vi "220428_snipper_v15.vi"(0 "Input picture 3":picture caption="Input", 1 "hh:mm:ss":T2={"left"=50, "top"=439, "right"=600, "bottom"=479} caption="input hh:mm:ss") -> (2 "4-bit pixmap":u8[][][](array[numeric]), 3 "sniped pic.":picture[](array[picture]), 4 "String N":i32, 5 "elapsed time(s)":dbl[][](array[numeric]) format="%#_3g")   [LabVIEW 2016]
panel:
  in  "Read data":bool
  out "Sumtime(s)":dbl
  out "From_TapN":dbl
  out "moveLog(Row, Col.) 2":i32[][](array[numeric])
  out "from TotalP 2":i32
  out "Out signal 2":bool
  out "From_TapN 2":dbl
  in  "N1 test(Col.)":i32
  in  "タブ制御器":T1(tab)
  out "Input picture":picture caption="Input"
  out "Void potition":cluster{"Y":dbl[], "Y":dbl[]}[](graph)
  out "Graph data":i32[][](array[numeric])
  out "Rawdata pixmap":u8[][](array[numeric]) caption="4ビットピックスマップ"
  in  "path to PNG file":path=path "G:/マイドライブ/STEPN/STEPN_walking/PNG/220510-220515/IMG_6679.PNG" caption="PNGファイルパス"
  out "Debug test pic. 4":picture caption="12 delete pic."
  out "Expand test pic. 5":picture caption="12 delete Expand pic."
  out "string(start,end) 2":i32[][](array[numeric])
  out "Debug test pic. 2":picture caption="7x pic."
  out "7x move(min, max)":i32[][](array[numeric])
  out "searchCol.by7x":i32[](array[numeric])
  out "ΔmoveLog(Row, Col.)":i32[][][](array[numeric])
  out "Debug test pic. 3":picture caption="Δ  pic."
  out "deruta bitmap":i32[][](array[numeric])
  out "OK/NG":string[][](array[string])
  out "Δ N":i32
  out "7xMove Log":i32[][][](array[numeric])
  out "NG_moveLog(Row, Col.)出力":i32[][][](array[numeric])
  out "OutPut_moveLog_all 2":i32[][][](array[numeric])
  out "2forward moveLog 2":i32[][][](array[numeric])
  out "7x Expand pic.":picture
  out "Δ Expand pic.":picture
  out "2F Expand pic.":picture
  out "pixmap size(T×Y)":i32[](array[numeric])
  out "Debug test pic.":picture caption="Debug naname pic."
  out "4-bit pixmap 3":u8[][](array[numeric])
  out "string 2":string[](array[string])
  out "To:finish Col. 2":i32
  out "to Total point 2":i32
  out "Left_TotalP 2":i32
  out "R_endCol. 2":i32
  out "L_endCol. 2":i32
  out "Debug test pic. 8":picture caption="Debug test pic."
  out "2forwardN 2":i32
  out "Right(1) or Left(2) 2":enum16{"1>2", "1=2", "1<2"}(ring)
  out "To(1) or From(2) 2":enum16{"1>2", "1=2", "1<2"}(ring)
  out "2forward totalP 2":i32[](array[numeric])
  out "Goal 2":i32
  out "from\\to 2":string
  out "Right_TotalP 2":i32
  out "Expand test pic. 2":picture caption="Debug naname pic."
  out "naname":bool
  out "Pixture size (Y, X)":i32[](array[numeric])
  out "naname_TotalP":i32
  out "TapN":dbl
  in  "naname hide":bool=TRUE
  out "4 detected":bool
  out "2F Expand pic. 2":picture caption="2F Expand pic."
  out "Δ Expand pic. 2":picture caption="Δ Expand Pic."
  out "2F Expand pic. 3":picture caption="2F Expand pic."
  out "R_TapN 2":dbl
  out "L_TapN 2":dbl
  out "Debug test pic. 6":picture caption="Debug test pic."
  out "Debug test pic. 7":picture caption="Debug test pic."
  out "Debug test pic. 5":picture caption="Debug test pic."
  in  "N1_test":bool
  # "v12 : 35/5(文字1のy/x) で切り取り\nv13 : 2段階①35/5で切り取り /一旦一区切り\n　　　　　　　　  ②2forward search(4を踏んだ時点で中断)"
  # "sec"
  # "%"
  # "0"
  # "1"
  # "2"
  # "3"
  # "4"
  # "5"
  # "6"
  # "7"
  # "Picture"
  # "File"
  # "OFF"
  # "ON"
  # "2forward : Yellow\nΔ　：Green"
  # "Left : blue\nTo : red"
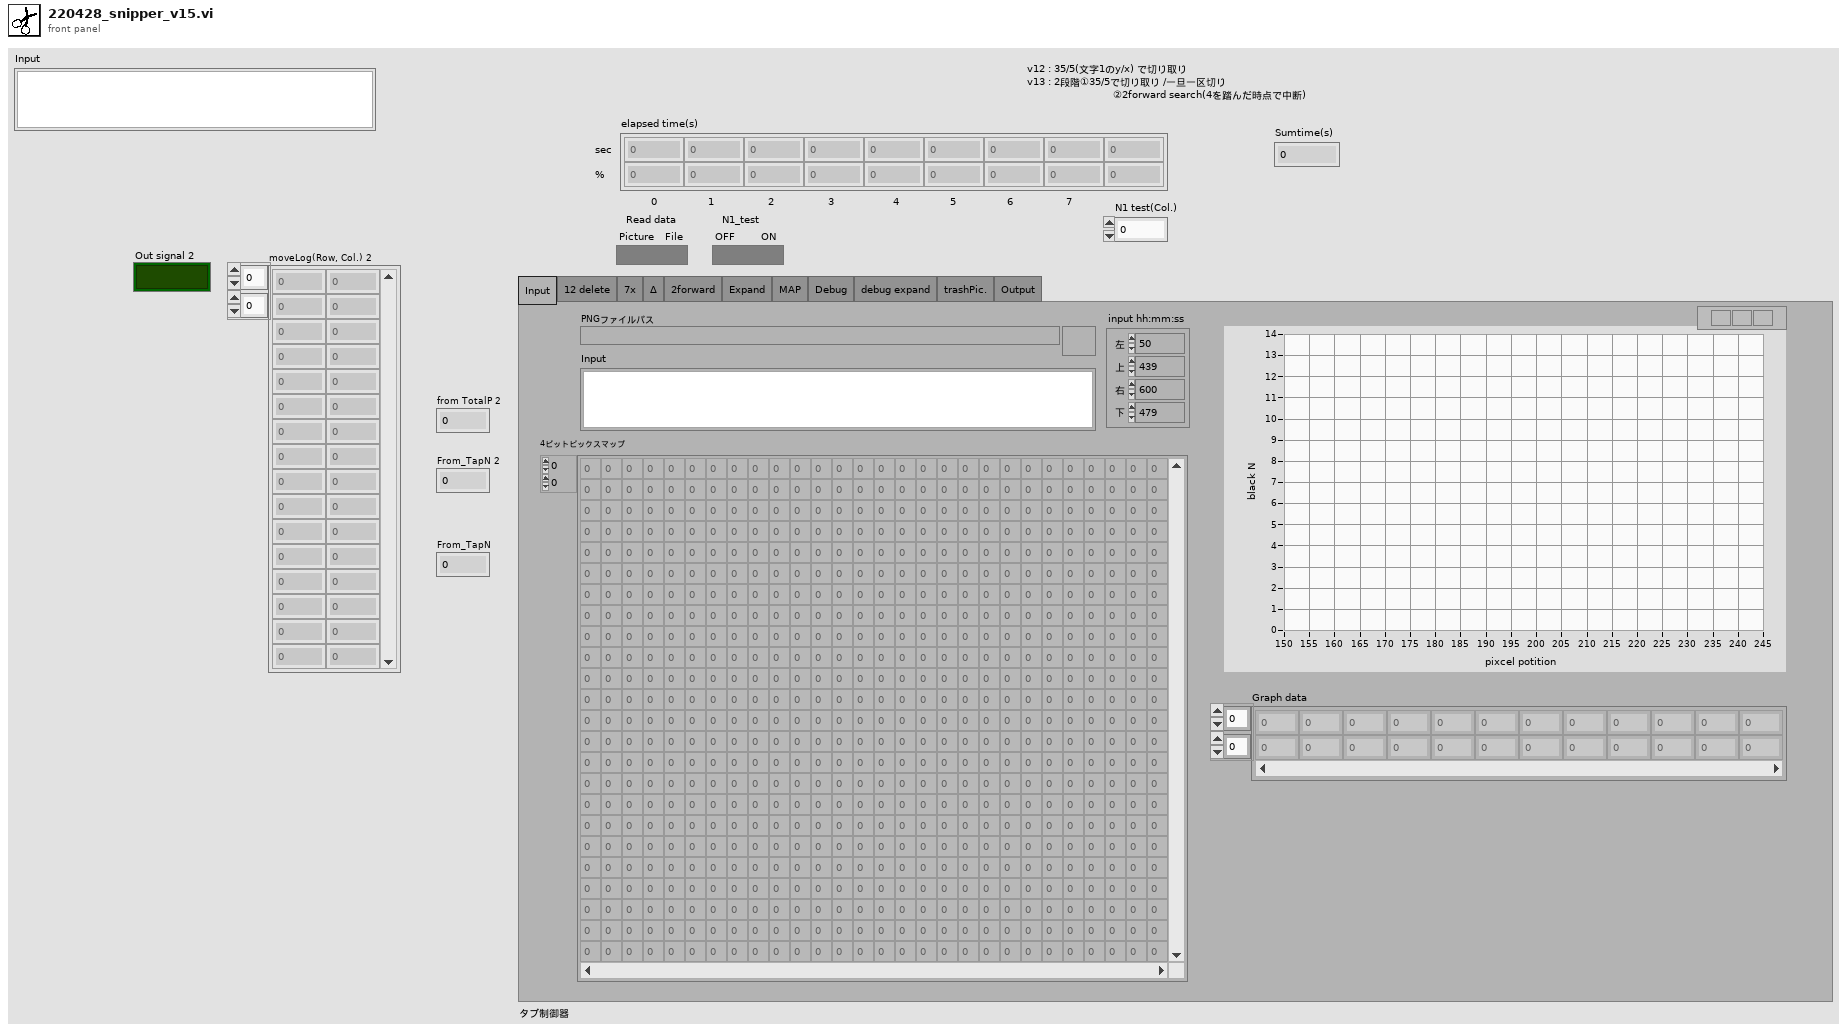
[diagram p1: front panel]
types:
  T1 = enum32{"Input", "12 delete", "7x", "Δ", "2forward", "Expand", "MAP", "Debug", "debug expand", "trashPic.", "Output"}
  T2 = cluster{"left":i16, "top":i16, "right":i16, "bottom":i16}
  T3 = typedef "imagedata.ctl" = cluster{"image type":i32, "image depth":i32, "image":u8[], "mask":u8[], "colors":u32[], "Rectangle":cluster{"left":i16, "top":i16, "right":i16, "bottom":i16}}
  T4 = typedef "LVBoundsTypeDef.ctl" = cluster{"Width":u32, "Height":u32}
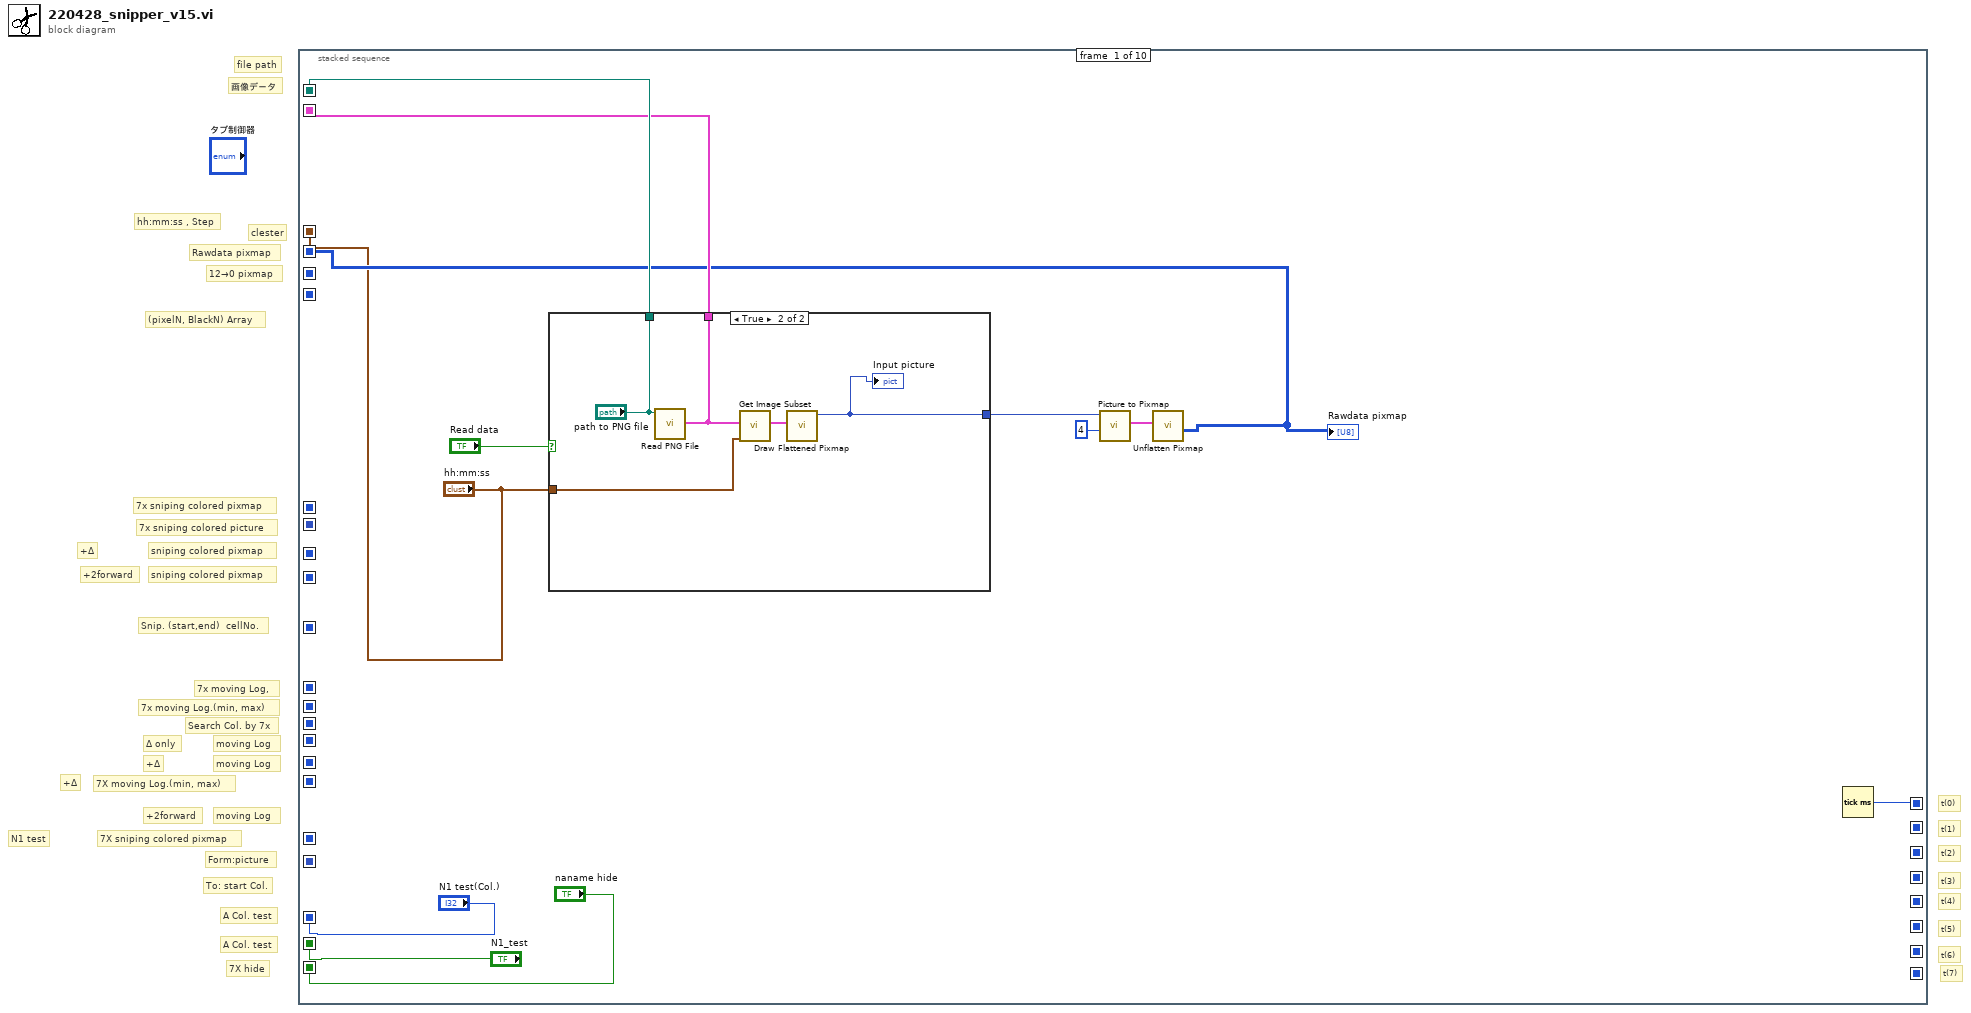
[diagram p0: block diagram]
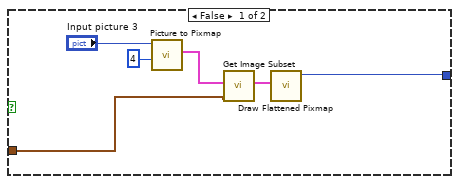
[diagram p2: hidden frame]
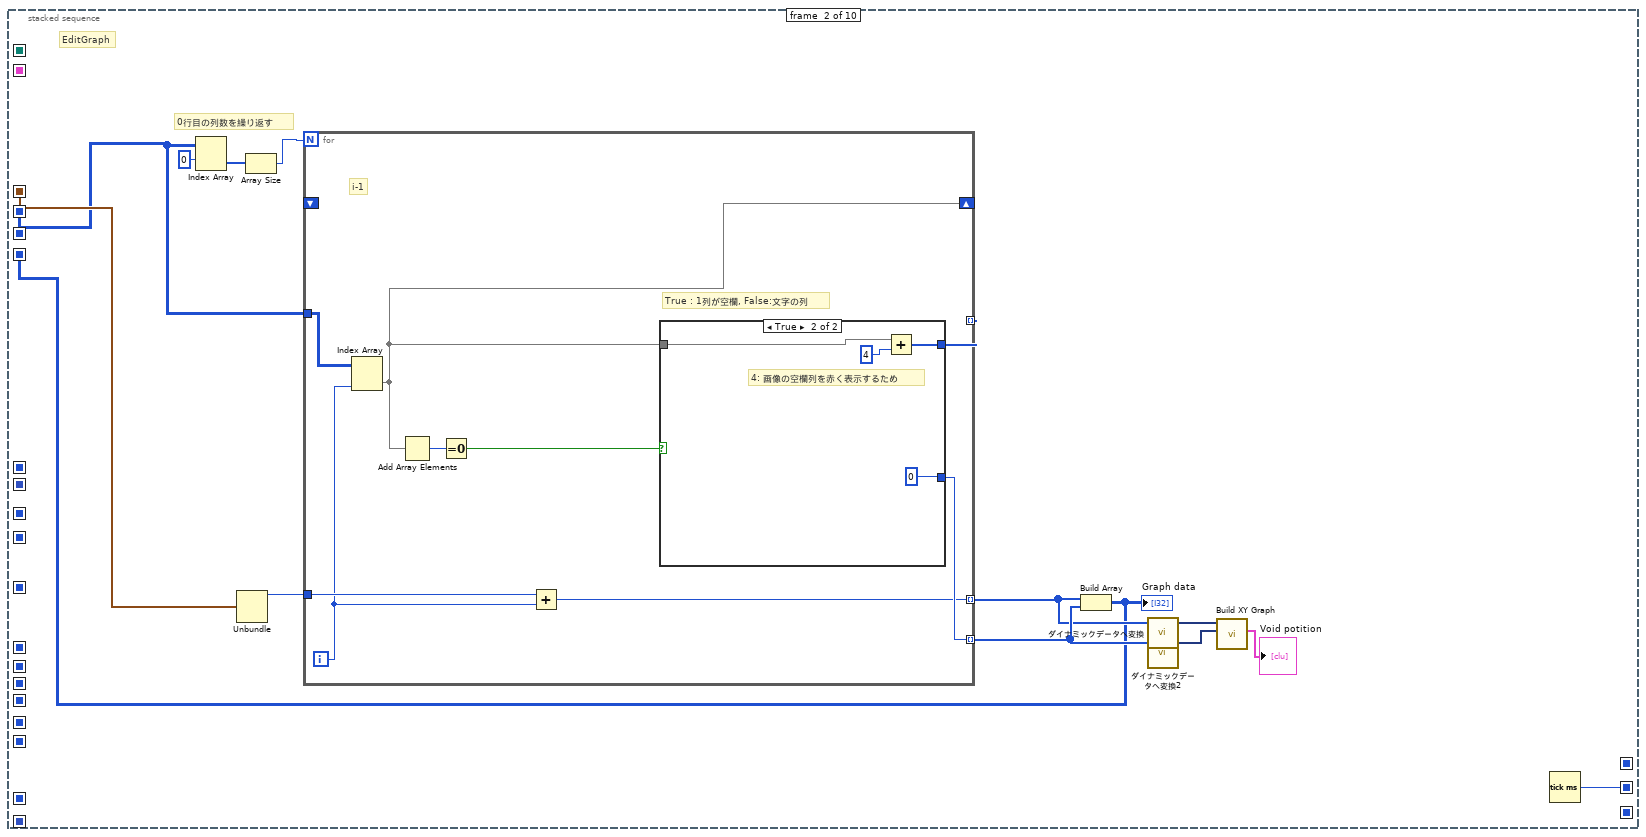
[diagram p3: hidden frame]
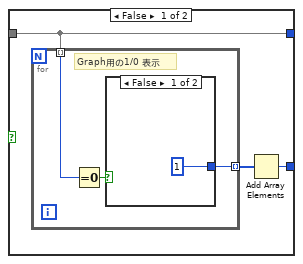
[diagram p4: hidden frame]
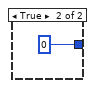
[diagram p5: hidden frame]
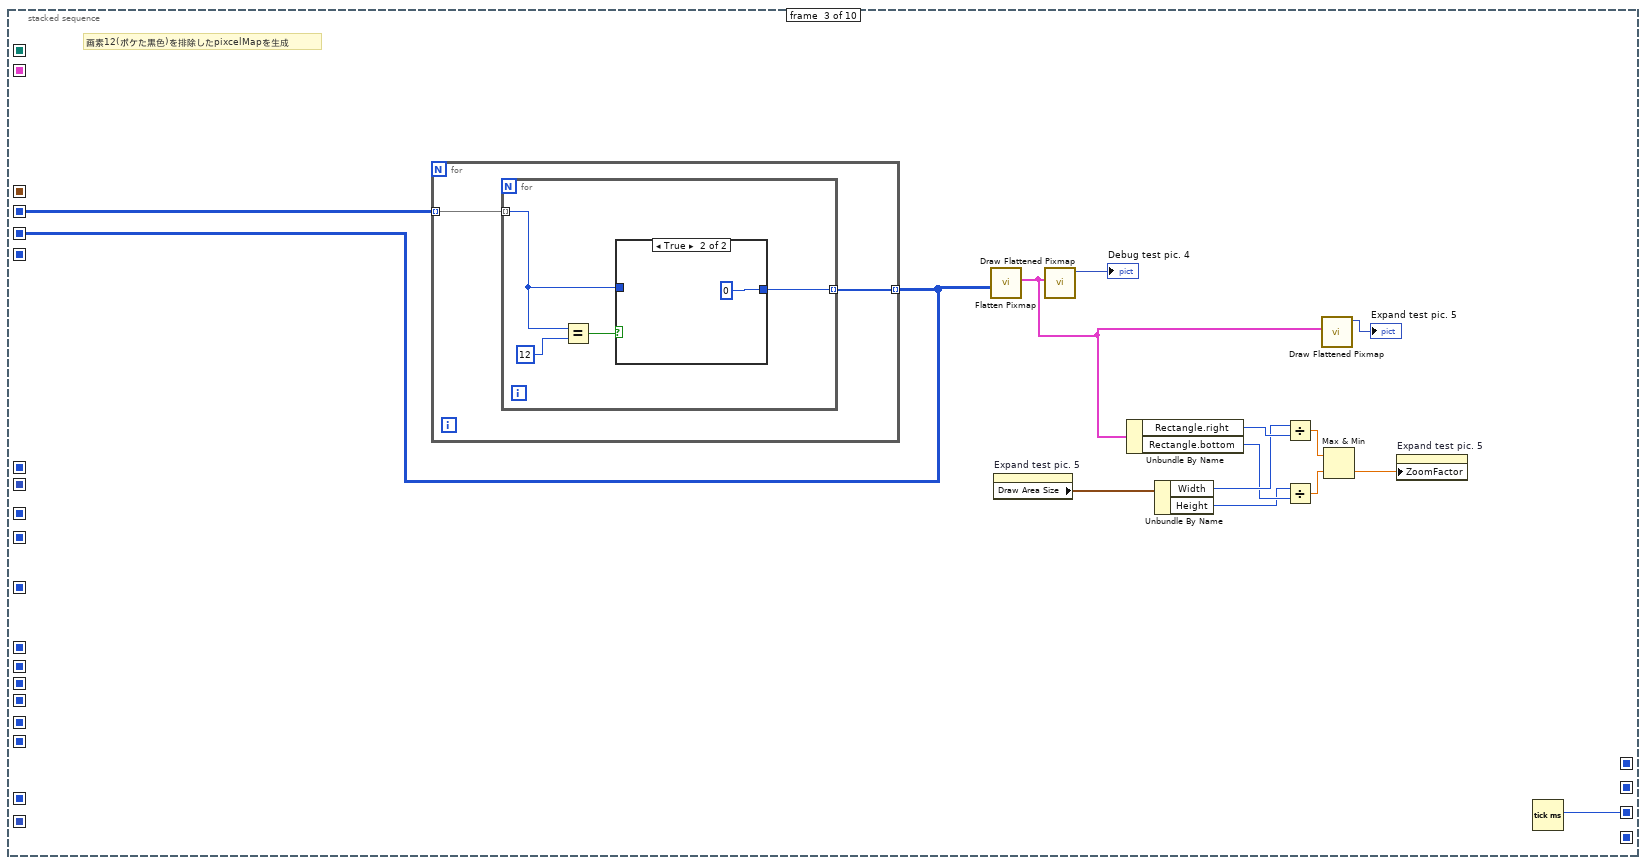
[diagram p6: hidden frame]
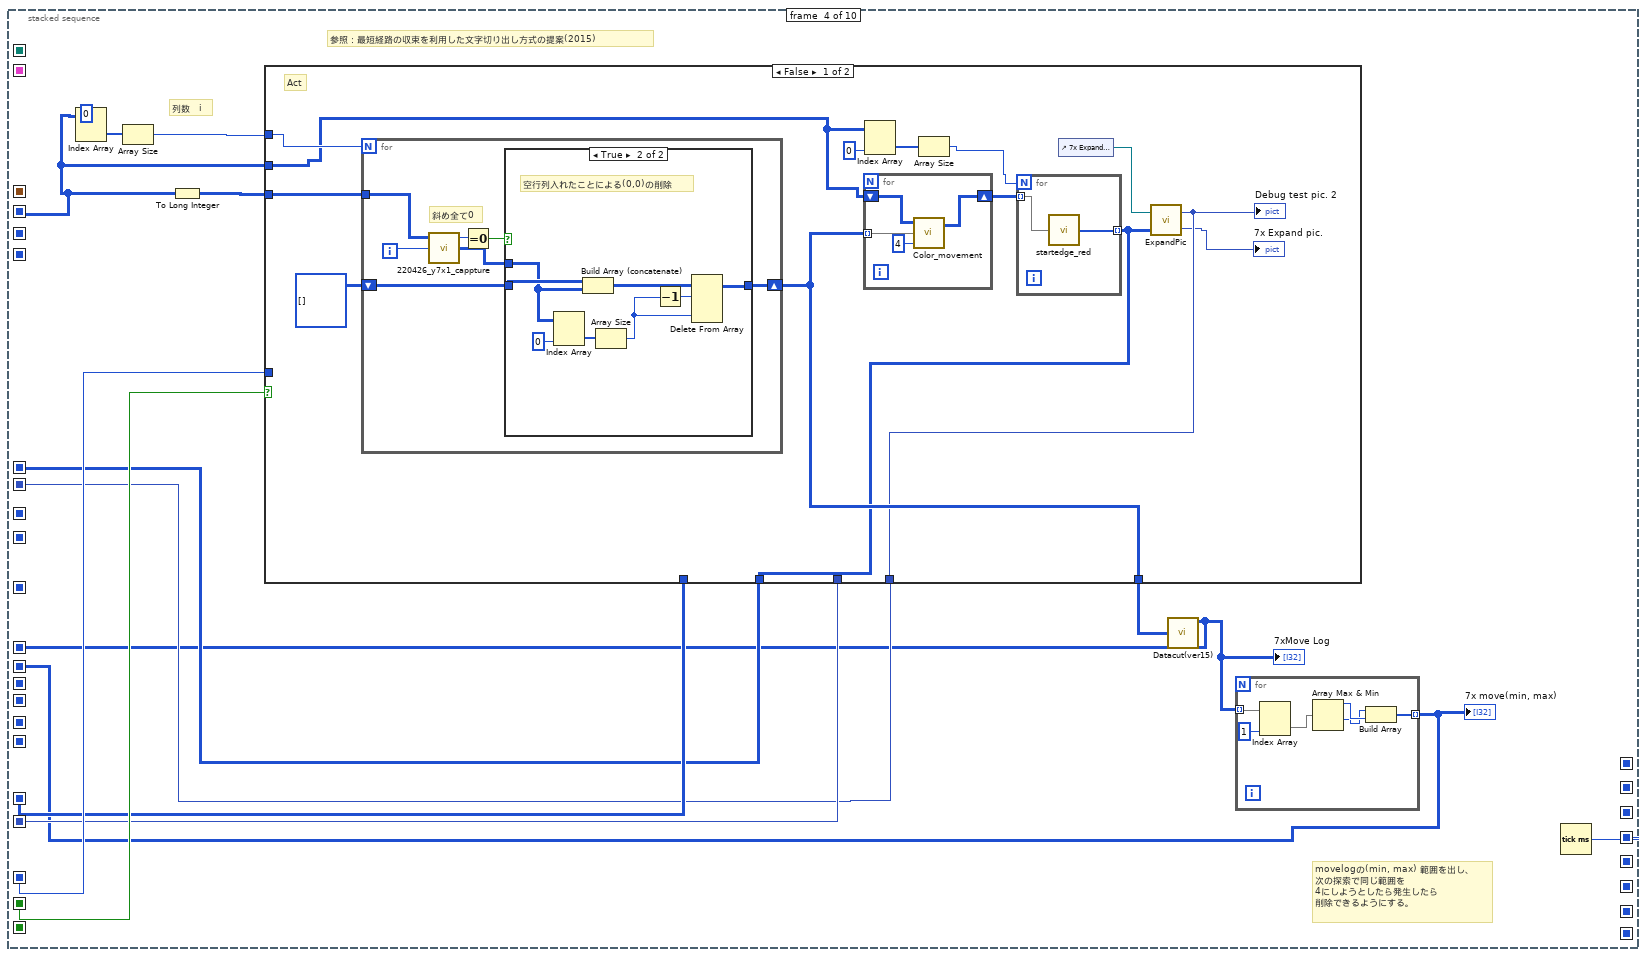
[diagram p8: hidden frame]
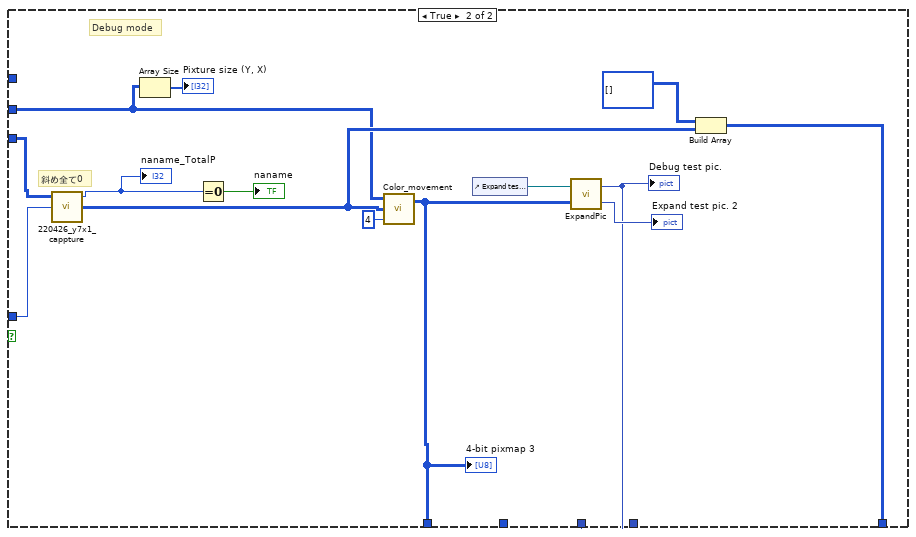
[diagram p10: hidden frame]
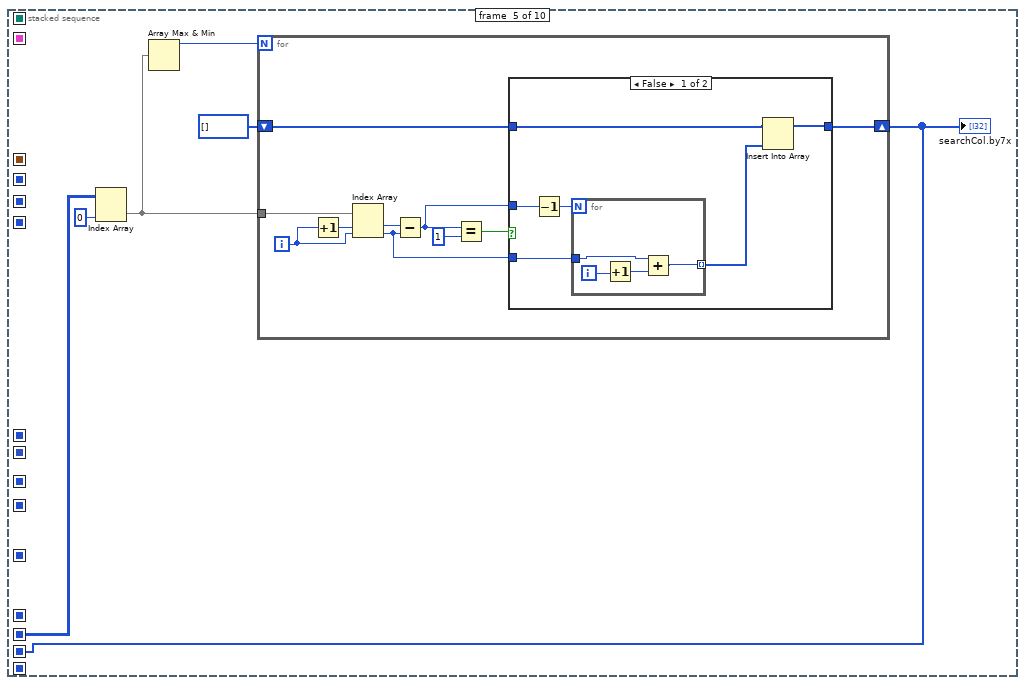
[diagram p11: hidden frame]
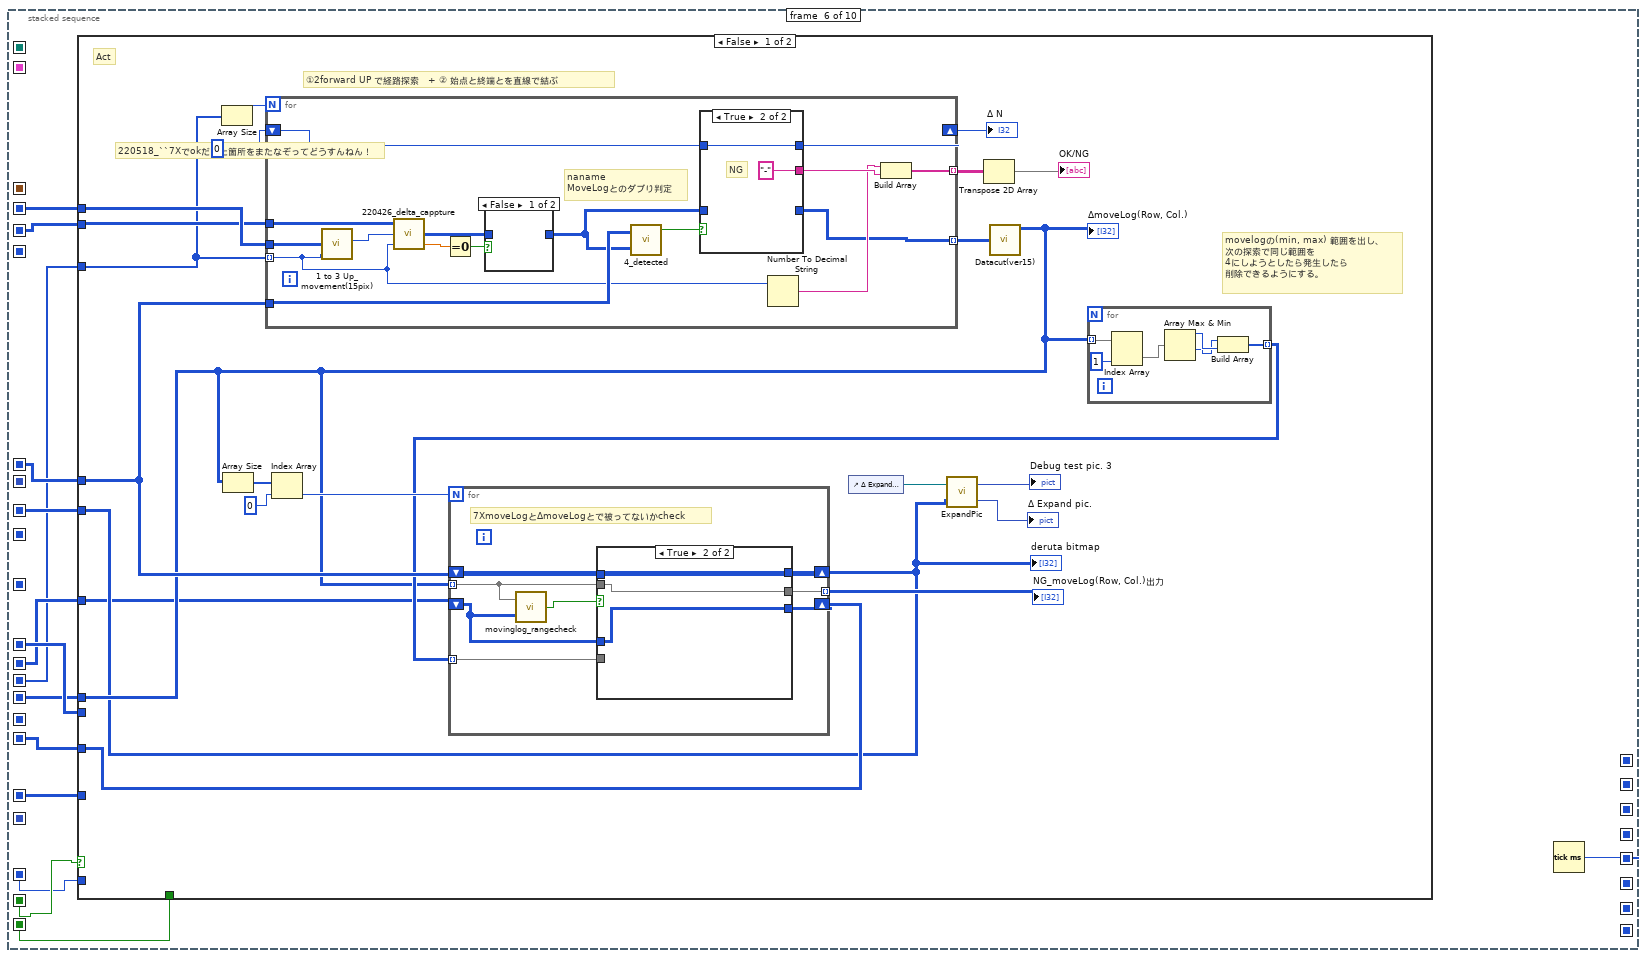
[diagram p13: hidden frame]
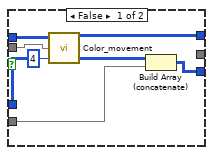
[diagram p14: hidden frame]
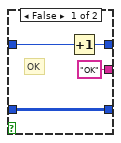
[diagram p15: hidden frame]
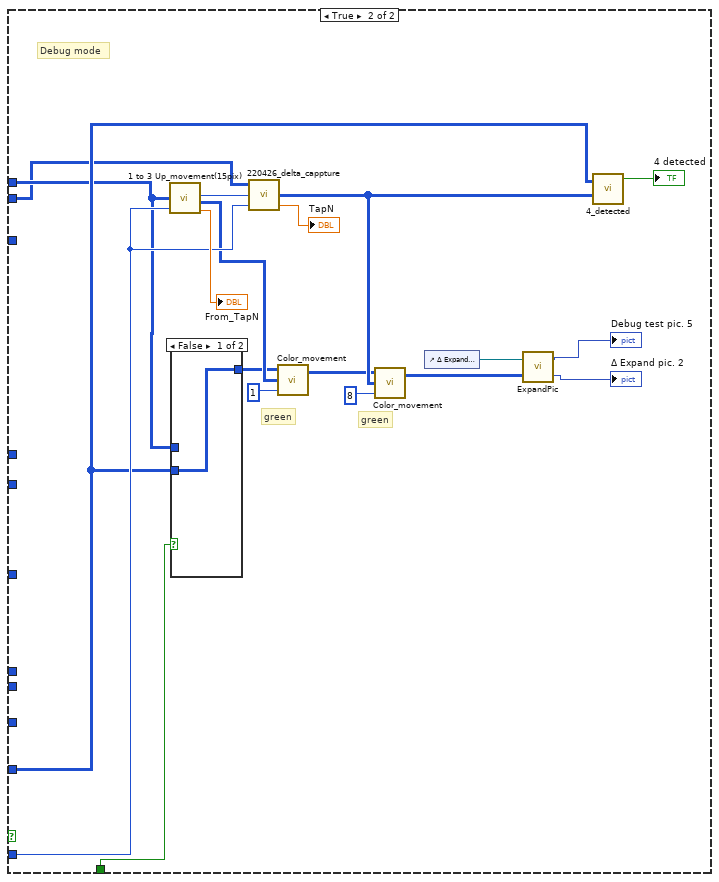
[diagram p17: hidden frame]
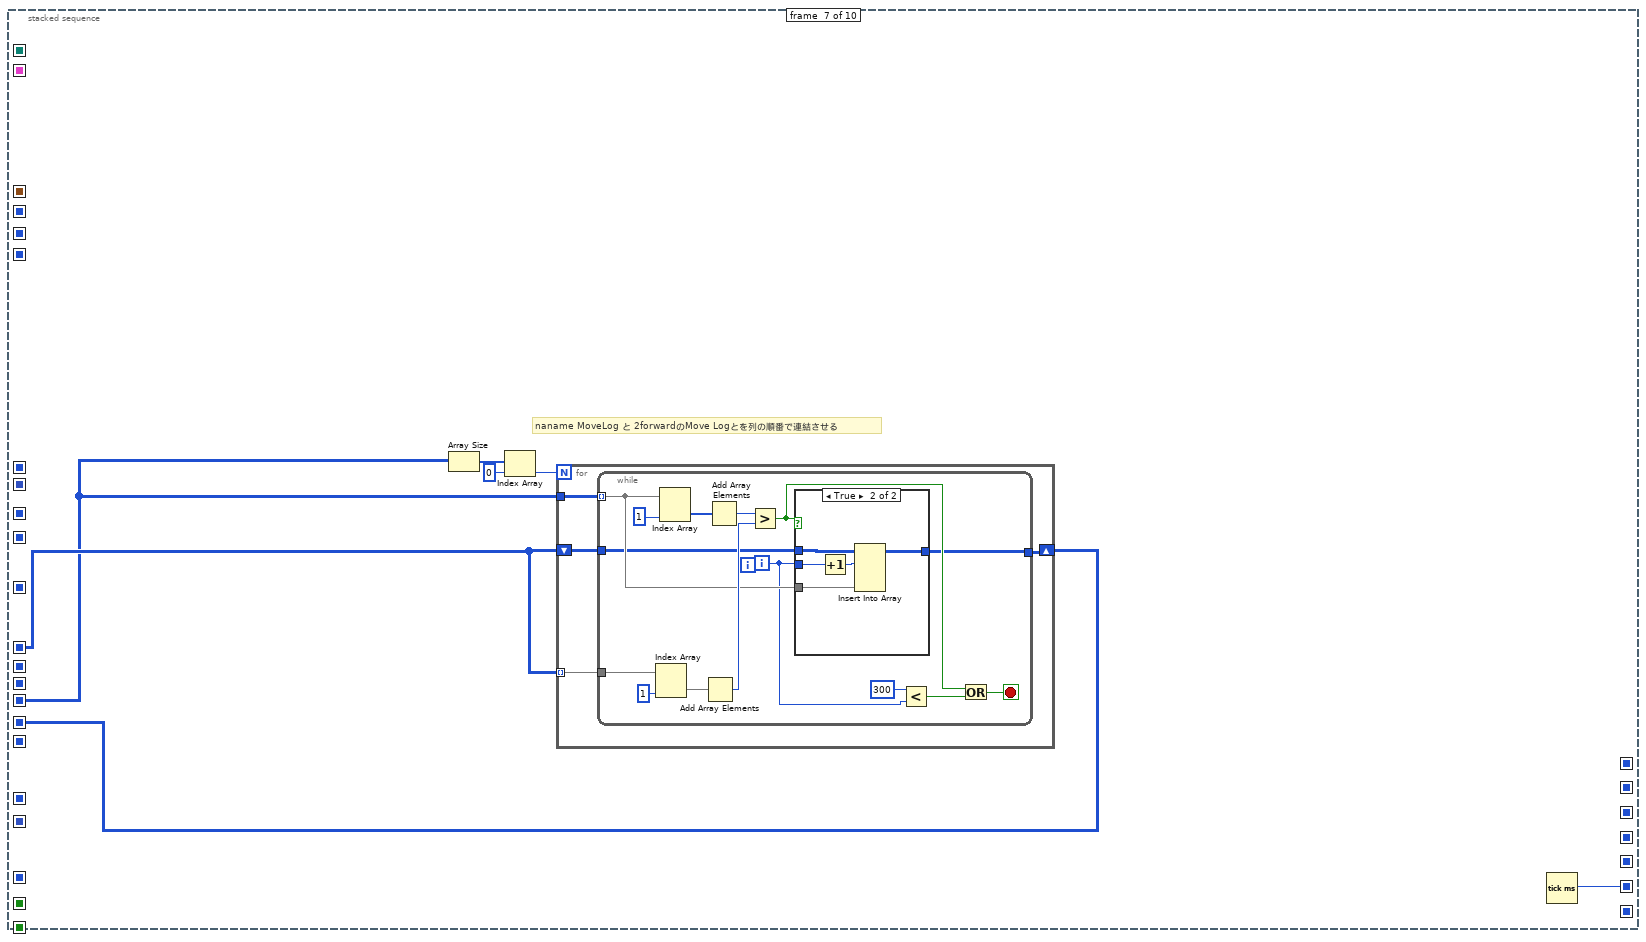
[diagram p19: hidden frame]
diagram:
  # "Search Col. by 7x"
  # "t(7)"
  # "Δ only"
  # "moving Log"
  # "7X moving Log.(min, max)"
  # "+Δ"
  # "t(6)"
  # "t(5)"
  # "t(4)"
  # "t(3)"
  # "t(2)"
  # "t(1)"
  # "7x moving Log.(min, max)"
  # "7X hide"
  # "+2forward"
  # "moving Log"
  # "+2forward"
  # "sniping colored pixmap"
  # "+Δ"
  # "moving Log"
  # "+Δ"
  # "7X sniping colored pixmap"
  # "7x sniping colored picture"
  # "t(0)"
  # "sniping colored pixmap"
  # "7x sniping colored pixmap"
  # "7x moving Log,"
  # "To: start Col."
  # "N1 test"
  # "Form:picture"
  # "A Col. test"
  # "A Col. test"
  # "画像データ"
  # "Snip. (start,end)  cellNo."
  # "(pixelN, BlackN) Array"
  # "12→0 pixmap"
  # "Rawdata pixmap"
  # "hh:mm:ss , Step"
  # "clester"
  # "file path"
  n1 = stacked-sequence {
    seq-local: [w12 _ _ _ _ _ _ _ _ _] -> [_ _ _ _ _ _ _ _ _ _]
    seq-local: ["hh:mm:ss" _ _ _ _ _ _ _ _ _] -> [_ w36 _ _ _ _ _ _ _ _]
    seq-local: [w6 _ _ _ _ _ _ _ _ _] -> [_ w27 w71 w84 _ w178 _ _ _ _]
    seq-local: [_ w25 _ _ _ _ _ _ _ _] -> [_ _ _ _ _ _ _ _ _ _]
    seq-local: [_ _ _ _ _ _ _ _ w496 _] -> [_ _ _ _ _ _ _ _ _ w541]
    seq-local: [w9 _ _ _ _ _ _ _ _ _] -> [_ _ _ _ _ _ _ _ _ _]
    seq-local: ["N1_test" _ _ _ _ _ _ _ _ _] -> [_ _ _ w92 _ w190 _ w323 _ _]
    seq-local: ["N1 test(Col.)" _ _ _ _ _ _ _ _ _] -> [_ _ _ w91 _ w189 _ w322 _ _]
    seq-local: [_ _ _ w90 _ _ _ _ _ _] -> [_ _ _ _ _ w188 _ w321 _ _]
    seq-local: [_ _ _ w89 _ _ _ _ _ _] -> [_ _ _ _ _ _ _ _ _ _]
    seq-local: [_ _ _ w81 _ _ _ _ _ _] -> [_ _ _ _ _ w187 w284 _ _ _]
    seq-local: [_ _ _ w86 _ _ _ _ _ _] -> [_ _ _ _ _ w186 _ _ _ _]
    seq-local: [_ _ _ _ _ _ _ w317 _ _] -> [_ _ _ _ _ _ _ _ w491 _]
    seq-local: [w5 _ _ _ _ _ _ _ _ _] -> [_ _ _ _ _ _ _ _ _ w521]
    seq-local: [_ _ _ w85 _ _ _ _ _ _] -> [_ _ _ _ _ _ _ _ _ _]
    seq-local: [_ _ _ _ _ _ w282 _ _ _] -> [_ _ _ _ _ _ _ w316 _ _]
    seq-local: [_ _ w58 _ _ _ _ _ _ _] -> [_ _ _ _ _ w185 _ w320 _ _]
    seq-local: [_ _ _ _ _ w184 _ _ _ _] -> [_ _ _ _ _ _ _ w315 _ w535]
    seq-local: ["naname hide" _ _ _ _ _ _ _ _ _] -> [_ _ _ _ _ w183 _ w319 _ _]
    seq-local: [_ _ _ w82 _ _ _ _ _ _] -> [_ _ _ _ w155 w182 _ _ _ _]
    seq-local: [_ w24 _ _ _ _ _ _ _ _] -> [_ _ _ _ _ _ _ _ _ w534]
    seq-local: [_ _ w70 _ _ _ _ _ _ _] -> [_ _ _ _ _ _ _ _ _ w533]
    seq-local: [_ _ _ w80 _ _ _ _ _ _] -> [_ _ _ _ _ _ _ _ _ w532]
    seq-local: [_ _ _ _ _ w181 _ _ _ _] -> [_ _ _ _ _ _ _ _ _ w531]
    seq-local: [_ _ _ _ _ _ w281 _ _ _] -> [_ _ _ _ _ _ _ _ _ w530]
    seq-local: [_ _ _ _ _ _ _ w314 _ _] -> [_ _ _ _ _ _ _ _ _ w529]
    seq-local: [_ _ _ _ _ w180 _ _ _ _] -> [_ _ _ _ _ _ _ w318 _ _]
    seq-local: [_ _ _ _ _ w179 _ _ _ _] -> [_ _ _ _ _ _ w283 _ _ _]
    seq-local: [_ _ _ _ _ _ _ _ w490 _] -> [_ _ _ _ _ _ _ _ _ w520]
    seq-local: [_ _ _ _ w150 _ _ _ _ _] -> [_ _ _ _ _ w177 _ w313 _ _]
    frame #0 {
      n2 = case shown="True" "Read data" {
        tunnel: [_ "path to PNG file"] -> w12
        tunnel: [_ w21] -> w9
        tunnel: [w13 w19] -> w3
        tunnel: "hh:mm:ss" -> [w17 w20]
        frame False {
          n3 = call <vilib>:"Picture to Pixmap.vi"("depth"=4, "picture"="Input picture 3") -> ("image data"=w14:T3)  [unwired: 8 in, 1 out]
          n4 = call <vilib>:"Get Image Subset.vi"("subset rect"=w17, "image data"=w14) -> ("image subset"=w18:T3)  [unwired: 4 in, 1 out]
          n5 = call <vilib>:"Draw Flattened Pixmap.vi"("image data"=w18) -> ("new picture"=w13:picture)  [unwired: 8 in]
        }
        frame True {
          n6 = call <vilib>:"Read PNG File.vi"("path to PNG file"="path to PNG file") -> ("image data"=w21:T3)  [unwired: 8 in, 2 out]
          n7 = call <vilib>:"Get Image Subset.vi"("subset rect"=w20, "image data"=w21) -> ("image subset"=w22:T3)  [unwired: 4 in, 1 out]
          n8 = call <vilib>:"Draw Flattened Pixmap.vi"("image data"=w22) -> ("new picture"=w19:picture)  [unwired: 8 in]
          "Input picture" <- w19
        }
      }
      n9 = call <vilib>:"Picture to Pixmap.vi"("depth"=4, "picture"=w3) -> ("image data"=w11:T3)  [unwired: 8 in, 1 out]
      n10 = call <vilib>:"Unflatten Pixmap.vi"("image data"=w11) -> ("4-bit pixmap"=w6:u8[][])  [unwired: 4 in, 6 out]
      "Rawdata pixmap" <- w6
      n11 = Tick Count (ms)() -> (millisecond timer value=w5:u32)
    }
    frame #1 {
      # "EditGraph"
      # "0行目の列数を繰り返す"
      n12 = Index Array(array=w27, index (row)=0) -> (element=w28:u8[])  [unwired: 1 in]
      n13 = Unbundle(w36) -> ("left"=w26:i16)  [unwired: 3 out]
      n14 = Array Size(array=w28) -> (size(s)=w29:i32)
      n15 = for {
        N: w29 -> [_]
        tunnel: w27 -> [w45]
        tunnel: [w38] -> w34 mode=indexing
        tunnel: w26 -> [w42]
        tunnel: [w39] -> w35 mode=indexing
        tunnel: [w40] -> _ mode=indexing
        shift-right: [w37] -> _
        shift-left: _ -> [_]
        i -> [w41]
        # "i-1"
        # "True : 1列が空欄, False:文字の列"
        n16 = Index Array(array=w45, index (col)=w41) -> (element=w37:u8[])  [unwired: 1 in]
        n17 = Add Array Elements(numeric array=w37) -> (sum=w43:u8)
        n18 = Equal To 0?(x=w43) -> (x = 0?=w44:bool)
        n19 = Add(x=w42, y=w41) -> (x+y=w38:i32)
        n20 = case shown="True" w44 {
          tunnel: w37 -> [w47 w57]
          tunnel: [w47 w56] -> w40
          tunnel: [w48 0] -> w39
          frame False {
            n21 = for {
              tunnel: w47 -> [w50] mode=indexing
              tunnel: [w49] -> w46 mode=indexing
              # "Graph用の1/0 表示"
              n22 = Equal To 0?(x=w50) -> (x = 0?=w51:bool)
              n23 = case shown="False" w51 {
                tunnel: [1 0] -> w49
                frame False {
                }
                frame True {
                }
              }
            }
            n24 = Add Array Elements(numeric array=w46) -> (sum=w48:i32)
          }
          frame True {
            # "4: 画像の空欄列を赤く表示するため"
            n25 = Add(x=w57, y=4) -> (x+y=w56:i32[])
          }
        }
      }
      n26 = Build Array(w34, w35) -> (w25:i32[][])
      "Graph data" <- w25
      n27 = call "ダイナミックデータへ変換"("Array"=w34) -> ("Dynamic Data Type"=w31:dynamicdata)  [unwired: 3 in]
      n28 = call "ダイナミックデータへ変換2"("Array"=w35) -> ("Dynamic Data Type"=w32:dynamicdata)  [unwired: 3 in]
      n29 = call "Build XY Graph"("Y Input"=w32, "X Input"=w31) -> ("XY Graph"=→"Void potition":cluster{"Y":dbl[], "Y":dbl[]}[])  [unwired: 8 in, 1 out]
      n30 = Tick Count (ms)() -> (millisecond timer value=w24:u32)
    }
    frame #2 {
      # "画素12(ボケた黒色)を排除したpixcelMapを生成"
      n31 = for {
        tunnel: w71 -> [w73] mode=indexing
        tunnel: [w72] -> w58 mode=indexing
        n32 = for {
          tunnel: w73 -> [w75] mode=indexing
          tunnel: [w74] -> w72 mode=indexing
          n33 = Equal?(x=w75, y=12) -> (x = y?=w76:bool)
          n34 = case shown="True" w76 {
            tunnel: w75 -> [w78 _]
            tunnel: [w78 0] -> w74
            frame False {
            }
            frame True {
            }
          }
        }
      }
      n35 = call <vilib>:"Flatten Pixmap.vi"("4-bit pixmap"=w58) -> ("image data"=w60:T3)  [unwired: 10 in]
      n36 = property on="Expand test pic. 5" class="Pict"() -> ("Draw Area Size"=w69:T4)  [unwired: 2 in, 2 out]
      n37 = call <vilib>:"Draw Flattened Pixmap.vi"("image data"=w60) -> ("new picture"=→"Debug test pic. 4":picture)  [unwired: 8 in]
      n38 = Unbundle By Name(w60) -> ("Rectangle.right"=w68:i16, "Rectangle.bottom"=w66:i16)
      n39 = Unbundle By Name(w69) -> ("Width"=w67:u32, "Height"=w65:u32)
      n40 = Divide(x=w67, y=w68) -> (x/y=w63:dbl)
      n41 = Divide(x=w65, y=w66) -> (x/y=w64:dbl)
      n42 = call <vilib>:"Draw Flattened Pixmap.vi"("image data"=w60) -> ("new picture"=→"Expand test pic. 5":picture)  [unwired: 8 in]
      n43 = Max & Min(x=w63, y=w64) -> (min(x,y)=w62:dbl)  [unwired: 1 out]
      n44 = property on="Expand test pic. 5" class="Pict"("ZoomFactor"=w62) -> ()  [unwired: 2 in, 2 out]
      n45 = Tick Count (ms)() -> (millisecond timer value=w70:u32)
    }
    frame #3 {
      # "movelogの(min, max) 範囲を出し、\n次の探索で同じ範囲を\n4にしようとしたら発生したら\n削除できるようにする。"
      # "参照：最短経路の収束を利用した文字切り出し方式の提案(2015)"
      # "列数　i"
      n46 = Index Array(array=w84, index (row)=0 ("指標")) -> (element=w93:u8[])  [unwired: 1 in]
      n47 = Array Size(array=w93) -> (size(s)=w88:i32)
      n48 = To Long Integer(number=w84) -> (32bit integer=w87:i32[][])
      n49 = case shown="False" w92 {
        tunnel: w88 -> [w111 _]
        tunnel: w87 -> [w113 w142]
        tunnel: [w109 w149] -> w83
        tunnel: w91 -> [_ w140]
        tunnel: [_ w139] -> w90
        tunnel: [_ w136] -> w89
        tunnel: [w104 _] -> w86
        tunnel: [w103 _] -> w85
        tunnel: w84 -> [w105 w141]
        frame False {
          # "Act"
          n50 = for {
            N: w111 -> [_]
            tunnel: w113 -> [w121]
            shift-right: [w122] -> w109
            shift-left: i32[][][] [] -> [w126]
            i -> [w120]
            # "斜め全て0"
            n51 = call "220426_y7x1_cappture.vi"("start Col."=w120, "Rawdata pixmap"=w121) -> ("moving Log(Y, X)"=w124:i32[][], "Total point"=w125:i32)  [unwired: 1 in, 1 out]
            n52 = Equal To 0?(x=w125) -> (x = 0?=w123:bool)
            n53 = case shown="True" w123 {
              tunnel: w126 -> [w127 w135]
              tunnel: [w127 w134] -> w122
              tunnel: w124 -> [_ w133]
              frame False {
              }
              frame True {
                # "空行列入れたことによる(0,0)の削除"
                n54 = Index Array(array=w133, index (col)=0 ("無効な指標 （列）")) -> (element=w130:i32[])  [unwired: 1 in]
                n55 = Build Array (concatenate)(w135, w133) -> (w132:i32[][][])
                n56 = Array Size(array=w130) -> (size(s)=w128:i32)
                n57 = Decrement(x=w128) -> (x-1=w129:i32)
                n58 = Delete From Array(array=w132, length=w129, index (dim 1)=w128) -> (array with subset deleted=w134:i32[][][])  [unwired: 2 in, 1 out]
              }
            }
          }
          n59 = for {
            tunnel: w109 -> [w119] mode=indexing
            shift-right: [w116] -> w110
            shift-left: w105 -> [w117]
            n60 = call "Color_movement.vi"("Color Number"=u8 4, "moveLog(Row, Col.)"=w119, "bitmap"=w117) -> ("Colored bitmap"=w116:i32[][])  [unwired: 1 in]
          }
          n61 = Index Array(array=w105, index (col)=0 ("無効な指標 （列）")) -> (element=w107:u8[])  [unwired: 1 in]
          n62 = Array Size(array=w107) -> (size(s)=w106:i32)
          n63 = for {
            N: w106 -> [_]
            tunnel: w110 -> [w115] mode=indexing
            tunnel: [w114] -> w104 mode=indexing
            n64 = call "startedge_red.vi"("4-bit pixmap入力"=w115) -> ("4-bit pixmap出力"=w114:u8[])
          }
          n65 = control-ref of="7x Expand pic."() -> (w102:refnum<vi>)
          n66 = call "ExpandPic.vi"("Colored bitmap"=w104, "Picture in"=w102) -> ("Expand test pic. 2"=→"7x Expand pic.":picture, "Debug test pic."=w103:picture)
          "Debug test pic. 2" <- w103
        }
        frame True {
          # "斜め全て0"
          # "Debug mode"
          n67 = call "220426_y7x1_cappture.vi"("start Col."=w140, "Rawdata pixmap"=w142) -> ("moving Log(Y, X)"=w144:i32[][], "Total point"=w147:i32)  [unwired: 1 in, 1 out]
          "naname_TotalP" <- w147
          n68 = Array Size(array=w141) -> (size(s)=→"Pixture size (Y, X)":i32[])
          n69 = Equal To 0?(x=w147) -> (x = 0?=→"naname":bool)
          n70 = call "Color_movement.vi"("Color Number"=u8 4, "moveLog(Row, Col.)"=w144, "bitmap"=w141) -> ("Colored bitmap"=w139:i32[][])  [unwired: 1 in]
          "4-bit pixmap 3" <- w139
          n71 = control-ref of="Expand test pic. 2"() -> (w138:refnum<vi>)
          n72 = call "ExpandPic.vi"("Colored bitmap"=w139, "Picture in"=w138) -> ("Expand test pic. 2"=→"Expand test pic. 2":picture, "Debug test pic."=w136:picture)
          "Debug test pic." <- w136
          n73 = Build Array(i32[][] [] ("要素"), w144) -> (w149:i32[][][])
        }
      }
      n74 = call "Datacut(ver15).vi"("moveLog(Row, Col.)入力"=w83) -> ("moveLog(Row, Col.)出力"=w81:i32[][][])  [unwired: 2 in, 3 out]
      "7xMove Log" <- w81
      n75 = for {
        tunnel: w81 -> [w97] mode=indexing
        tunnel: [w98] -> w82 mode=indexing
        n76 = Index Array(array=w97, index (col)=1 ("無効な指標 （列）")) -> (element=w95:i32[])  [unwired: 1 in]
        n77 = Array Max & Min(array=w95) -> (max value=w100:i32, min value=w99:i32)  [unwired: 2 out]
        n78 = Build Array(w99, w100) -> (w98:i32[])
      }
      "7x move(min, max)" <- w82
      n79 = Tick Count (ms)() -> (millisecond timer value=w80:u32)
    }
    frame #4 {
      n80 = Index Array(array=w155, index (col)=0 ("disabled index (col)")) -> (element=w152:i32[])  [unwired: 1 in]
      n81 = Array Max & Min(array=w152) -> (max value=w151:i32)  [unwired: 3 out]
      n82 = for {
        N: w151 -> [_]
        tunnel: w152 -> [w165]
        shift-right: [w158] -> w150
        shift-left: i32[] [] -> [w159]
        i -> [w164]
        n83 = Increment(x=w164) -> (x+1=w163:i32)
        n84 = Index Array(array=w165, index #1=w163, index #2=w164) -> (element #1=w162:i32, element #2=w156:i32)
        n85 = Subtract(x=w162, y=w156) -> (x-y=w157:i32)
        n86 = Equal?(x=w157, y=1) -> (x = y?=w161:bool)
        n87 = case shown="False" w161 {
          tunnel: w159 -> [w168 w176]
          tunnel: [w166 w176] -> w158
          tunnel: w157 -> [w170 _]
          tunnel: w156 -> [w169 _]
          frame False {
            n88 = Decrement(x=w170) -> (x-1=w171:i32)
            n89 = for {
              N: w171 -> [_]
              tunnel: w169 -> [w173]
              tunnel: [w172] -> w167 mode=indexing
              i -> [w175]
              n90 = Increment(x=w175) -> (x+1=w174:i32)
              n91 = Add(x=w173, y=w174) -> (x+y=w172:i32)
            }
            n92 = Insert Into Array(array=w168, new element=w167) -> (w166:i32[])  [unwired: 1 in]
          }
          frame True {
          }
        }
      }
      "searchCol.by7x" <- w150
    }
    frame #5 {
      n93 = case shown="False" w190 {
        tunnel: w189 -> [_ w276]
        tunnel: w188 -> [_ w271]
        tunnel: w185 -> [w197 w268]
        tunnel: [w195 _] -> w184
        tunnel: w187 -> [_ _]
        tunnel: w186 -> [w208 _]
        tunnel: w183 -> [_ w273]
        tunnel: w182 -> [w192 _]
        tunnel: [w200 _] -> w180
        tunnel: [w199 _] -> w179
        tunnel: w178 -> [w198 w269]
        tunnel: w177 -> [w191 _]
        frame False {
          # "220518_``7Xでokだった箇所をまたなぞってどうすんねん！"
          # "movelogの(min, max) 範囲を出し、\n次の探索で同じ範囲を\n4にしようとしたら発生したら\n削除できるようにする。"
          # "①2forward UP で経路探索　+ ② 始点と終端とを直線で結ぶ"
          # "Act"
          n94 = Array Size(array=w191) -> (size(s)=w212:i32)
          n95 = for {
            N: w212 -> [_]
            tunnel: w198 -> [w252]
            tunnel: w208 -> [w242]
            tunnel: [w241] -> w207 mode=indexing
            tunnel: [w248] -> w206 mode=indexing
            shift-right: [w243] -> w203
            shift-left: 0 -> [w240]
            tunnel: w197 -> [w238]
            tunnel: w191 -> [w237] mode=indexing
            # "naname\nMoveLogとのダブり判定"
            n96 = call "1 to 3 Up_movement(15pix).vi"("Input pixmap"=w252, "start Column"=w237) -> ("From:finish Col."=w244:i32)  [unwired: 1 in, 3 out]
            n97 = call "220426_delta_cappture.vi"("start Col."=w237, "end Col."=w244, "Rawdata pixmap"=w238) -> ("TapN"=w250:dbl, "moving Log(Y, X)"=w245:i32[][])  [unwired: 1 out]
            n98 = Equal To 0?(x=w250) -> (x = 0?=w251:bool)
            n99 = case shown="False" w251 {
              tunnel: [_ w259] -> w239
              tunnel: w245 -> [_ w259]
              frame False {
              }
              frame True {
              }
            }
            n100 = call "4_detected.vi"("4-bit pixmap"=w242, "moving Log(Row, Col.)"=w239) -> ("4 detected"=w249:bool)  [unwired: 1 in, 1 out]
            n101 = case shown="True" w249 {
              tunnel: [w256 _] -> w241
              tunnel: w239 -> [w256 _]
              tunnel: ["OK" "-"] -> w247
              tunnel: [w254 w257] -> w243
              tunnel: w240 -> [w253 w257]
              frame False {
                # "OK"
                n102 = Increment(x=w253) -> (x+1=w254:i32)
              }
              frame True {
                # "NG"
              }
            }
            n103 = Number To Decimal String(number=w237) -> (decimal integer string=w246:string)  [unwired: 1 in]
            n104 = Build Array(w246, w247) -> (w248:string[])
          }
          "Δ N" <- w203
          n105 = control-ref of="Δ Expand pic."() -> (w196:refnum<vi>)
          n106 = Transpose 2D Array(2D array=w206) -> (transposed array=→"OK/NG":string[][])
          n107 = call "Datacut(ver15).vi"("moveLog(Row, Col.)入力"=w207) -> ("moveLog(Row, Col.)出力"=w199:i32[][][])  [unwired: 2 in, 3 out]
          "ΔmoveLog(Row, Col.)" <- w199
          n108 = Array Size(array=w199) -> (size(s)=w210:i32[])
          n109 = Index Array(array=w210, index=0 ("指標")) -> (element=w211:i32)
          n110 = for {
            tunnel: w199 -> [w215] mode=indexing
            tunnel: [w216] -> w201 mode=indexing
            n111 = Index Array(array=w215, index (col)=1 ("無効な指標 （列）")) -> (element=w213:i32[])  [unwired: 1 in]
            n112 = Array Max & Min(array=w213) -> (max value=w218:i32, min value=w217:i32)  [unwired: 2 out]
            n113 = Build Array(w217, w218) -> (w216:i32[])
          }
          n114 = for {
            N: w211 -> [_]
            tunnel: w199 -> [w224] mode=indexing
            shift-right: [w226] -> w195
            shift-left: w208 -> [w225]
            tunnel: [w222] -> w202 mode=indexing
            shift-right: [w219] -> w200
            shift-left: w192 -> [w221]
            tunnel: w201 -> [w220] mode=indexing
            # "7XmoveLogとΔmoveLogとで被ってないかcheck"
            n115 = call "movinglog_rangecheck.vi"("naname movingLog(min, max)"=w221, "ΔmoveLog(Row, Col.)"=w224) -> ("daburi"=w223:bool)
            n116 = case shown="True" w223 {
              tunnel: [w232 w236] -> w226
              tunnel: w225 -> [w231 w236]
              tunnel: w224 -> [w230 w235]
              tunnel: [_ w235] -> w222
              tunnel: w221 -> [w229 w234]
              tunnel: w220 -> [w228 _]
              tunnel: [w227 w234] -> w219
              frame False {
                n117 = call "Color_movement.vi"("Color Number"=u8 4, "moveLog(Row, Col.)"=w230, "bitmap"=w231) -> ("Colored bitmap"=w232:i32[][])  [unwired: 1 in]
                n118 = Build Array (concatenate)(w229, w228) -> (w227:i32[][])
              }
              frame True {
              }
            }
          }
          "deruta bitmap" <- w195
          "NG_moveLog(Row, Col.)出力" <- w202
          n119 = call "ExpandPic.vi"("Colored bitmap"=w195, "Picture in"=w196) -> ("Expand test pic. 2"=→"Δ Expand pic.":picture, "Debug test pic."=→"Debug test pic. 3":picture)
        }
        frame True {
          # "green"
          # "green"
          # "Debug mode"
          n120 = call "1 to 3 Up_movement(15pix).vi"("Input pixmap"=w269, "start Column"=w276) -> ("From:finish Col."=w275:i32, "moveLog(Row, Col.)"=w266:i32[][], "TapN"=→"From_TapN":dbl)  [unwired: 1 in, 1 out]
          n121 = case shown="False" w273 {
            tunnel: w269 -> [_ w280]
            tunnel: w271 -> [w279 _]
            tunnel: [w279 w280] -> w265
            frame False {
            }
            frame True {
            }
          }
          n122 = call "220426_delta_cappture.vi"("start Col."=w276, "end Col."=w275, "Rawdata pixmap"=w268) -> ("TapN"=→"TapN":dbl, "moving Log(Y, X)"=w272:i32[][])  [unwired: 1 out]
          n123 = call "Color_movement.vi"("Color Number"=u8 1, "moveLog(Row, Col.)"=w266, "bitmap"=w265) -> ("Colored bitmap"=w264:i32[][])  [unwired: 1 in]
          n124 = call "Color_movement.vi"("Color Number"=u8 8, "moveLog(Row, Col.)"=w272, "bitmap"=w264) -> ("Colored bitmap"=w262:i32[][])  [unwired: 1 in]
          n125 = control-ref of="Δ Expand pic. 2"() -> (w263:refnum<vi>)
          n126 = call "ExpandPic.vi"("Colored bitmap"=w262, "Picture in"=w263) -> ("Expand test pic. 2"=→"Δ Expand pic. 2":picture, "Debug test pic."=→"Debug test pic. 5":picture)
          n127 = call "4_detected.vi"("4-bit pixmap"=w271, "moving Log(Row, Col.)"=w272) -> ("4 detected"=→"4 detected":bool)  [unwired: 1 in, 1 out]
        }
      }
      n128 = Tick Count (ms)() -> (millisecond timer value=w181:u32)
    }
    frame #6 {
      # "naname MoveLog と 2forwardのMove Logとを列の順番で連結させる"
      n129 = Array Size(array=w283) -> (size(s)=w287:i32[])
      n130 = Index Array(array=w287, index=0 ("指標")) -> (element=w285:i32)
      n131 = for {
        N: w285 -> [_]
        tunnel: w284 -> [w291] mode=indexing
        tunnel: w283 -> [w290]
        shift-right: [w289] -> w282
        shift-left: w284 -> [w288]
        n132 = while {
          tunnel: w291 -> [w306]
          tunnel: w290 -> [w299] mode=indexing
          tunnel: [w293] -> w289
          tunnel: w288 -> [w292]
          i -> [w297]
          stop <- w294 stop-if-true
          n133 = Index Array(array=w306, index (col)=1 ("無効な指標 （列）")) -> (element=w304:i32[])  [unwired: 1 in]
          n134 = Index Array(array=w299, index (col)=1 ("無効な指標 （列）")) -> (element=w301:i32[])  [unwired: 1 in]
          n135 = Add Array Elements(numeric array=w304) -> (sum=w303:i32)
          n136 = Add Array Elements(numeric array=w301) -> (sum=w302:i32)
          n137 = Greater?(x=w302, y=w303) -> (0:w295:bool)
          n138 = case shown="True" w295 {
            tunnel: w292 -> [w307 w312]
            tunnel: w297 -> [_ w310]
            tunnel: w299 -> [_ w309]
            tunnel: [w307 w308] -> w293
            frame False {
            }
            frame True {
              n139 = Increment(x=w310) -> (x+1=w311:i32)
              n140 = Insert Into Array(array=w312, index (dim 0)=w311, new element=w309) -> (w308:i32[][][])  [unwired: 2 in]
            }
          }
          n141 = Less?(x=300, y=w297) -> (x < y?=w296:bool)
          n142 = Or(x=w295, y=w296) -> (x .or. y?=w294:bool)
        }
      }
      n143 = Tick Count (ms)() -> (millisecond timer value=w281:u32)
    }
    frame #7 {
      n144 = case shown="False" w323 {
        tunnel: w322 -> [_ w459]
        tunnel: w321 -> [_ w472]
        tunnel: w320 -> [w336 w451]
        tunnel: w316 -> [w344 _]
        tunnel: w315 -> [w335 _]
        tunnel: [w329 _] -> w317
        tunnel: w319 -> [_ w450]
        tunnel: w315 -> [w333 _]
        tunnel: w318 -> [w331 _]
        tunnel: w313 -> [w324 _]
        frame False {
          # "naname MoveLog と 2forwardのMove Logとを列の順番で連結させる"
          # "Act"
          # "2forward N"
          # "Capture N"
          # "切り分け箇所を赤で可視化"
          n145 = Array Size(array=w324) -> (size(s)=w325:i32)
          n146 = for {
            N: w325 -> [_]
            tunnel: [w416] -> w343 mode=indexing
            tunnel: [w415] -> w342 mode=indexing
            shift-right: [w413] -> w348
            shift-left: 0 -> [w414]
            tunnel: w335 -> [w412]
            tunnel: w336 -> [w411]
            tunnel: [w409] -> w338 mode=indexing
            tunnel: [w392] -> w334 mode=indexing
            tunnel: w324 -> [w385] mode=indexing
            # "Tap≧4"
            # "4をふんだらOUT"
            # "fromの出発と\n toの着地"
            # "Totalpoint 小さい方"
            n147 = call "1 to 3 Up_movement(15pix).vi"("Input pixmap"=w411, "start Column"=w385) -> ("Total point"=w418:i32, "From:finish Col."=w419:i32, "moveLog(Row, Col.)"=w417:i32[][], "TapN"=w410:dbl)  [unwired: 1 in]
            n148 = call "1 to 3 Down_movement_v11.vi"("Input pixmap"=w411, "start Column"=w419) -> ("Total point"=w406:i32, "moveLog(Row, Col.)"=w405:i32[][], "To:finish Col."=w404:i32, "TapN"=w403:dbl)  [unwired: 1 in]
            n149 = call "1 to 3 Down_movement_v12.vi"("Input pixmap"=w411, "start Column"=w419) -> ("Total point"=w402:i32, "moveLog(Row, Col.)"=w401:i32[][], "To:finish Col."=w400:i32, "TapN"=w399:dbl)  [unwired: 1 in]
            n150 = call "Tap_valuation.vi"("1st_Col."=w404, "1st_moveLog"=w405, "1st_TotalP"=w406, "1st_TapN"=w403, "2nd_TotalP"=w402, "2nd_moveLog"=w401, "2nd Col."=w400, "2nd_TapN"=w399, "start Col."=w385) -> ("1st or 2nd"=→"Right(1) or Left(2) 2":enum16{"1>2", "1=2", "1<2"}, "Out_TotalP"=w398:i32, "Out_TapN"=w397:dbl, "OutPut_moveLog"=w396:i32[][], "Out_ Col."=w395:i32)  [unwired: 2 in]
            n151 = Equal?(x=w395, y=w385) -> (x = y?=w408:bool)
            n152 = case shown="True" w408 {
              tunnel: w418 -> [_ w432]
              tunnel: w417 -> [_ w431]
              tunnel: [_ w428] -> w407
              tunnel: [_ w429] -> w392
              tunnel: w398 -> [_ w436]
              tunnel: w397 -> [_ w435]
              tunnel: w396 -> [_ w434]
              tunnel: w395 -> [_ w433]
              tunnel: w410 -> [_ w430]
              tunnel: w385 -> [_ w426]
              tunnel: [_ w427] -> w386
              frame False {
              }
              frame True {
                # "from or to"
                n153 = call "Tap_valuation.vi"("1st_Col."=w433, "1st_moveLog"=w434, "1st_TotalP"=w436, "1st_TapN"=w435, "2nd_TotalP"=w432, "2nd_moveLog"=w431, "2nd Col."=w426, "2nd_TapN"=w430, "start Col."=w426) -> ("Out_TotalP"=w428:i32, "OutPut_moveLog"=w429:i32[][], "Out_ Col."=w427:i32)  [unwired: 2 in, 2 out]
              }
            }
            "To(1) or From(2) 2" <- w386
            n154 = call "4_detected.vi"("4-bit pixmap"=w412, "moving Log(Row, Col.)"=w392) -> ("4 detected"=w390:bool, "tapN"=w388:i32)  [unwired: 1 in]
            n155 = Number To Decimal String(number=w386) -> (decimal integer string=w393:string)  [unwired: 1 in]
            n156 = Greater Or Equal?(x=w388, y=5) -> (x >= y?=w387:bool)
            n157 = Or(x=w390, y=w387) -> (x .or. y?=w391:bool)
            n158 = case shown="True" w391 {
              tunnel: [w424 _] -> w415
              tunnel: w407 -> [w424 _]
              tunnel: [w421 _] -> w416
              tunnel: w392 -> [w421 _]
              tunnel: w414 -> [w423 w425]
              tunnel: [w422 w425] -> w413
              tunnel: w393 -> [w420 _]
              tunnel: [w420 _] -> w409
              frame False {
                n159 = Increment(x=w423) -> (x+1=w422:i32)
              }
              frame True {
              }
            }
          }
          "2forwardN 2" <- w348
          "OutPut_moveLog_all 2" <- w334
          n160 = control-ref of="2F Expand pic."() -> (w330:refnum<vi>)
          n161 = call "Datacut(ver15).vi"("Input Total P"=w342, "moveLog(Row, Col.)入力"=w343, "Input 1st or 2nd"=w338) -> ("moveLog(Row, Col.)出力"=w326:i32[][][], "Output Total P"=→"2forward totalP 2":i32[], "Input 1st or 2nd 2"=→"string 2":string[])  [unwired: 1 out]
          "2forward moveLog 2" <- w326
          n162 = Array Size(array=w326) -> (size(s)=w340:i32[])
          n163 = Index Array(array=w340, index=0 ("指標")) -> (element=w332:i32)
          n164 = for {
            N: w332 -> [_]
            tunnel: w326 -> [w352] mode=indexing
            shift-right: [w354] -> w329
            shift-left: w333 -> [w353]
            tunnel: w331 -> [w350]
            # "今回のΔmoveLogと被ってないかcheck"
            n165 = call "movinglog_rangecheck.vi"("naname movingLog(min, max)"=w350, "ΔmoveLog(Row, Col.)"=w352) -> ("daburi"=w351:bool)
            n166 = case shown="False" w351 {
              tunnel: [w357 w359] -> w354
              tunnel: w353 -> [w356 w359]
              tunnel: w352 -> [w355 _]
              frame False {
                n167 = call "Color_movement.vi"("Color Number"=u8 4, "moveLog(Row, Col.)"=w355, "bitmap"=w356) -> ("Colored bitmap"=w357:i32[][])  [unwired: 1 in]
              }
              frame True {
              }
            }
          }
          n168 = call "ExpandPic.vi"("Colored bitmap"=w329, "Picture in"=w330) -> ("Expand test pic. 2"=→"2F Expand pic.":picture, "Debug test pic."=→"Debug test pic. 6":picture)
          n169 = Array Size(array=w326) -> (size(s)=w347:i32[])
          n170 = Index Array(array=w347, index=0 ("指標")) -> (element=w345:i32)
          n171 = for {
            N: w345 -> [_]
            tunnel: w344 -> [w363] mode=indexing
            tunnel: w326 -> [w362]
            shift-right: [w361] -> _
            shift-left: w344 -> [w360]
            n172 = while {
              tunnel: w363 -> [w378]
              tunnel: w362 -> [w371] mode=indexing
              tunnel: [w365] -> w361
              tunnel: w360 -> [w364]
              i -> [w369]
              stop <- w366 stop-if-true
              n173 = Index Array(array=w378, index (col)=1 ("無効な指標 （列）")) -> (element=w376:i32[])  [unwired: 1 in]
              n174 = Index Array(array=w371, index (col)=1 ("無効な指標 （列）")) -> (element=w373:i32[])  [unwired: 1 in]
              n175 = Add Array Elements(numeric array=w376) -> (sum=w375:i32)
              n176 = Add Array Elements(numeric array=w373) -> (sum=w374:i32)
              n177 = Greater?(x=w374, y=w375) -> (0:w367:bool)
              n178 = case shown="True" w367 {
                tunnel: w364 -> [w379 w384]
                tunnel: w369 -> [_ w382]
                tunnel: w371 -> [_ w381]
                tunnel: [w379 w380] -> w365
                frame False {
                }
                frame True {
                  n179 = Increment(x=w382) -> (x+1=w383:i32)
                  n180 = Insert Into Array(array=w384, index (dim 0)=w383, new element=w381) -> (w380:i32[][][])  [unwired: 2 in]
                }
              }
              n181 = Less?(x=300, y=w369) -> (x < y?=w368:bool)
              n182 = Or(x=w367, y=w368) -> (x .or. y?=w366:bool)
            }
          }
        }
        frame True {
          # "Tap≧4"
          # "red"
          # "blue"
          # "green"
          # "4をふんだらOUT"
          # "優先順位：\n①：文字を踏んだ回数\n②：Totalpoint"
          # "Debug mode"
          n183 = call "1 to 3 Up_movement(15pix).vi"("Input pixmap"=w451, "start Column"=w459) -> ("Total point"=w466:i32, "From:finish Col."=w461:i32, "moveLog(Row, Col.)"=w467:i32[][], "TapN"=w457:dbl)  [unwired: 1 in]
          "from TotalP 2" <- w466
          "From_TapN 2" <- w457
          n184 = case shown="True" w450 {
            tunnel: w451 -> [_ w482]
            tunnel: [w481 w482] -> w455
            tunnel: w472 -> [w481 _]
            frame False {
            }
            frame True {
            }
          }
          n185 = call "1 to 3 Down_movement_v11.vi"("Input pixmap"=w451, "start Column"=w461) -> ("Total point"=w469:i32, "moveLog(Row, Col.)"=w453:i32[][], "To:finish Col."=w471:i32, "TapN"=w470:dbl)  [unwired: 1 in]
          "Right_TotalP 2" <- w469
          "R_endCol. 2" <- w471
          "R_TapN 2" <- w470
          n186 = call "1 to 3 Down_movement_v12.vi"("Input pixmap"=w451, "start Column"=w461) -> ("Total point"=w468:i32, "moveLog(Row, Col.)"=w452:i32[][], "To:finish Col."=w478:i32, "TapN"=w458:dbl)  [unwired: 1 in]
          "Left_TotalP 2" <- w468
          "L_endCol. 2" <- w478
          "L_TapN 2" <- w458
          n187 = call "Color_movement.vi"("Color Number"=u8 8, "moveLog(Row, Col.)"=w467, "bitmap"=w455) -> ("Colored bitmap"=w441:i32[][])  [unwired: 1 in]
          n188 = control-ref of="2F Expand pic. 2"() -> (w444:refnum<vi>)
          n189 = call "ExpandPic.vi"("Colored bitmap"=w441, "Picture in"=w444) -> ("Expand test pic. 2"=→"2F Expand pic. 2":picture, "Debug test pic."=→"Debug test pic. 7":picture)
          n190 = call "Tap_valuation.vi"("1st_Col."=w471, "1st_moveLog"=w453, "1st_TotalP"=w469, "1st_TapN"=w470, "2nd_TotalP"=w468, "2nd_moveLog"=w452, "2nd Col."=w478, "2nd_TapN"=w458, "start Col."=w459) -> ("Out_TotalP"=w462:i32, "Out_TapN"=w465:dbl, "OutPut_moveLog"=w463:i32[][], "Out_ Col."=w464:i32)  [unwired: 2 in, 1 out]
          "to Total point 2" <- w462
          "To:finish Col. 2" <- w464
          n191 = call "Tap_valuation.vi"("1st_Col."=w464, "1st_moveLog"=w463, "1st_TotalP"=w462, "1st_TapN"=w465, "2nd_TotalP"=w466, "2nd_moveLog"=w467, "2nd Col."=w461, "2nd_TapN"=w457, "start Col."=w459) -> ("OutPut_moveLog"=w460:i32[][])  [unwired: 2 in, 4 out]
          n192 = call "Color_movement.vi"("Color Number"=u8 3, "moveLog(Row, Col.)"=w453, "bitmap"=w455) -> ("Colored bitmap"=w454:i32[][])  [unwired: 1 in]
          n193 = Less Or Equal?(x=w462, y=w466) -> (x <= y?=w477:bool)
          n194 = call "Color_movement.vi"("Color Number"=u8 6, "moveLog(Row, Col.)"=w452, "bitmap"=w454) -> ("Colored bitmap"=w439:i32[][])  [unwired: 1 in]
          n195 = case shown="False" w477 {
            tunnel: w460 -> [w483 w486]
            tunnel: [w483 w486] -> w473
            tunnel: ["from" "to"] -> w476
            frame False {
            }
            frame True {
            }
          }
          "from\\to 2" <- w476
          n196 = control-ref of="2F Expand pic. 3"() -> (w440:refnum<vi>)
          n197 = call "ExpandPic.vi"("Colored bitmap"=w439, "Picture in"=w440) -> ("Expand test pic. 2"=→"2F Expand pic. 3":picture, "Debug test pic."=→"Debug test pic. 8":picture)
          n198 = call "4_detected.vi"("4-bit pixmap"=w451, "moving Log(Row, Col.)"=w473) -> ("4 detected"=w445:bool, "tapN"=w446:i32)  [unwired: 1 in]
          "Out signal 2" <- w445
          n199 = Greater Or Equal?(x=w446, y=5) -> (x >= y?=w448:bool)
          n200 = Or(x=w445, y=w448) -> (x .or. y?=w447:bool)
          n201 = case shown="True" w447 {
            tunnel: [w488 _] -> w475
            tunnel: w473 -> [w488 _]
            tunnel: [1 0] -> w479
            frame False {
            }
            frame True {
            }
          }
          "Goal 2" <- w479
          "moveLog(Row, Col.) 2" <- w475
        }
      }
      n202 = Tick Count (ms)() -> (millisecond timer value=w314:u32)
    }
    frame #8 {
      # "i行内における4と4の間の文字を切り取る"
      # "① N(i)=4, N(i-1) =4 → 何もしない\n② N(i)=文字, N(i-1) = 4 → pixel(i)を取得\n③ N(i)=文字, N(i-1) = 文字 → 何もしない\n④ N(i)=4, N(i-1) = 文字 → pixel(i-1)を取得"
      # "文字の開始端と終端を検出する"
      n203 = Index Array(array=w491, index (col)=0 ("無効な指標 （列）")) -> (element=w494:i32[])  [unwired: 1 in]
      n204 = Array Size(array=w494) -> (size(s)=w493:i32)
      n205 = for {
        N: w493 -> [_]
        tunnel: w491 -> [w503]
        tunnel: [w498] -> w492 mode=indexing
        i -> [w500]
        # "i-2列目"
        # "i-1列目"
        # "i列目"
        # "行の数を繰り返す"
        n206 = Index Array(array=w503, index (row)=w500) -> (element=w502:i32[])  [unwired: 1 in]
        n207 = for {
          tunnel: w502 -> [w508] mode=indexing
          tunnel: [w510] -> w499 mode=indexing
          shift-right: [w508] -> _
          shift-left: u8 4 -> [w504]
          shift-right: [w504] -> _
          shift-left: u8 4 -> [_]
          i -> [w505]
          w506 = 4
          # "True: 空欄の列、False: 文字の列"
          n208 = Equal?(x=w506, y=w508) -> (x = y?=w509:bool)
          n209 = Equal?(x=w506, y=w504) -> (x = y?=w507:bool)
          n210 = case shown="False" w509 {
            tunnel: w507 -> [w513 w517]
            tunnel: [w512 w515] -> w510
            tunnel: w505 -> [w511 w516]
            frame False {
              # "②,③"
              n211 = case shown="True" w513 {
                tunnel: [_ w514] -> w512
                tunnel: w511 -> [_ w514]
                frame False {
                  # "③"
                }
                frame True {
                  # "②"
                }
              }
            }
            frame True {
              # "①, ④"
              n212 = case shown="False" w517 {
                tunnel: [w518 _] -> w515
                tunnel: w516 -> [w519 _]
                frame False {
                  # "④"
                  n213 = Decrement(x=w519) -> (x-1=w518:i32)
                }
                frame True {
                  # "①"
                }
              }
            }
          }
        }
        n214 = call "DataCut(Ver.3).vi"("Input data array"=w499) -> ("Output data array"=w498:dbl[])
      }
      n215 = To Long Integer(number=w492) -> (32bit integer=w496:i32[][])
      "string(start,end) 2" <- w496
      n216 = Tick Count (ms)() -> (millisecond timer value=w490:u32)
    }
    frame #9 {
      # "列数/2(文字数)の数を繰り返す"
      n217 = Index Array(array=w541, index (row)=0 ("指標 （行）")) -> (element=w543:i32[])  [unwired: 1 in]
      n218 = Array Size(array=w543) -> (size(s)=w542:i32)
      n219 = Quotient & Remainder(x=w542, y=2) -> (floor(x/y)=w544:i32)  [unwired: 1 out]
      n220 = for {
        N: w544 -> [_]
        tunnel: w535 -> [w557]
        tunnel: w541 -> [w561]
        tunnel: [w554] -> w539 mode=indexing
        i -> [w553]
        # "i行目の文字を抽出"
        # "end"
        # "start"
        n221 = Multiply(x=2, y=w553) -> (x*y=w550:i32)
        n222 = Increment(x=w550) -> (x+1=w551:i32)
        n223 = Index Array(array=w561, index (col) #1=w550, index (col) #2=w551) -> (element #1=w555:i32[], element #2=w556:i32[])  [unwired: 2 in]
        n224 = Index Array(array=w557, index (col)=0 ("指標 （行）")) -> (element=w560:i32[])  [unwired: 1 in]
        n225 = Array Max & Min(array=w555) -> (min value=w563:i32)  [unwired: 3 out]
        n226 = Array Max & Min(array=w556) -> (max value=w562:i32)  [unwired: 3 out]
        n227 = Array Size(array=w560) -> (size(s)=w559:i32)
        n228 = for {
          N: w559 -> [_]
          tunnel: w563 -> [w566]
          tunnel: w562 -> [w569]
          tunnel: w557 -> [w571] mode=indexing
          tunnel: w556 -> [w568] mode=indexing
          tunnel: w555 -> [w565] mode=indexing
          tunnel: [w570] -> w554 mode=indexing
          # "T : そのまま範囲抽出, F: max,minの分を0で補正して範囲抽出"
          n229 = Equal?(x=w565, y=w566) -> (x = y?=w573:bool)
          n230 = Equal?(x=w568, y=w569) -> (x = y?=w572:bool)
          n231 = Subtract(x=w565, y=w566) -> (x-y=w564:i32)
          n232 = Subtract(x=w569, y=w568) -> (x-y=w567:i32)
          n233 = case shown="False" w573 {
            tunnel: w572 -> [w574 w618]
            tunnel: w571 -> [w579 w617]
            tunnel: [w580 w616] -> w570
            tunnel: w566 -> [w576 w615]
            tunnel: w569 -> [w577 w614]
            tunnel: w567 -> [w575 w613]
            tunnel: w564 -> [w578 _]
            frame False {
              n234 = case shown="False" w574 {
                tunnel: [w584 w608] -> w580
                tunnel: w579 -> [w591 w606]
                tunnel: w578 -> [w589 w605]
                tunnel: w577 -> [w590 w604]
                tunnel: w576 -> [w583 w603]
                tunnel: w575 -> [w586 _]
                frame False {
                  # "end"
                  n235 = Subtract(x=w590, y=w583) -> (x-y=w582:i32)
                  n236 = Increment(x=w582) -> (x+1=w581:i32)
                  n237 = Delete From Array(array=w591, length=w581, index=w583) -> (deleted portion=w592:i32[])  [unwired: 1 out]
                  n238 = for {
                    N: w589 -> [_]
                    shift-right: [w599] -> w588
                    shift-left: w592 -> [w600]
                    i -> [w598]
                    n239 = Replace Array Subset(array=w600, new element=0.0 ("新規要素/部分配列"), index=w598) -> (w599:i32[])
                  }
                  n240 = Reverse 1D Array(array=w588) -> (reversed array=w587:i32[])
                  n241 = for {
                    N: w586 -> [_]
                    shift-right: [w595] -> w585
                    shift-left: w587 -> [w596]
                    i -> [w594]
                    n242 = Replace Array Subset(array=w596, new element=0.0 ("新規要素/部分配列"), index=w594) -> (w595:i32[])
                  }
                  n243 = Reverse 1D Array(array=w585) -> (reversed array=w584:i32[])
                }
                frame True {
                  # "end"
                  n244 = Subtract(x=w604, y=w603) -> (x-y=w602:i32)
                  n245 = Increment(x=w602) -> (x+1=w601:i32)
                  n246 = Delete From Array(array=w606, length=w601, index=w603) -> (deleted portion=w607:i32[])  [unwired: 1 out]
                  n247 = for {
                    N: w605 -> [_]
                    shift-right: [w611] -> w608
                    shift-left: w607 -> [w612]
                    i -> [w610]
                    n248 = Replace Array Subset(array=w612, new element=0.0 ("新規要素/部分配列"), index=w610) -> (w611:i32[])
                  }
                }
              }
            }
            frame True {
              # "start"
              n249 = case shown="True" w618 {
                tunnel: w617 -> [w628 w638]
                tunnel: [w622 w637] -> w616
                tunnel: w615 -> [w621 w635]
                tunnel: w614 -> [w627 w636]
                tunnel: w613 -> [w625 _]
                frame False {
                  n250 = Subtract(x=w627, y=w621) -> (x-y=w620:i32)
                  n251 = Increment(x=w620) -> (x+1=w619:i32)
                  n252 = Delete From Array(array=w628, length=w619, index=w621) -> (deleted portion=w626:i32[])  [unwired: 1 out]
                  n253 = Reverse 1D Array(array=w626) -> (reversed array=w624:i32[])
                  n254 = for {
                    N: w625 -> [_]
                    shift-right: [w632] -> w623
                    shift-left: w624 -> [w631]
                    i -> [w630]
                    n255 = Replace Array Subset(array=w631, new element=u8 0 ("新規要素/部分配列"), index=w630) -> (w632:i32[])
                  }
                  n256 = Reverse 1D Array(array=w623) -> (reversed array=w622:i32[])
                }
                frame True {
                  n257 = Subtract(x=w636, y=w635) -> (x-y=w633:i32)
                  n258 = Increment(x=w633) -> (x+1=w634:i32)
                  n259 = Delete From Array(array=w638, length=w634, index=w635) -> (deleted portion=w637:i32[])  [unwired: 1 out]
                }
              }
            }
          }
        }
      }
      "4-bit pixmap" <- w539
      n260 = Array Size(array=w539) -> (size(s)=w537:i32[])
      "pixmap size(T×Y)" <- w537
      n261 = for {
        tunnel: [w548] -> w540 mode=indexing
        tunnel: w539 -> [w547] mode=indexing
        n262 = call <vilib>:"Flatten Pixmap.vi"("4-bit pixmap"=w547) -> ("image data"=w549:T3)  [unwired: 10 in]
        n263 = call <vilib>:"Draw Flattened Pixmap.vi"("image data"=w549) -> ("new picture"=w548:picture)  [unwired: 8 in]
      }
      "sniped pic." <- w540
      n264 = Index Array(array=w537, index=0 ("指標")) -> (element=→"String N":i32)
      n265 = Build Array(w521, w534, w533, w532, w531, w530, w529, w520) -> (w522:u32[])
      n266 = call "segment time.vi"("Intial time t(0)"=w521, "segment time t(i-1)"=w522) -> ("% time oqupied"=w528:dbl[], "segment time t(i)-t(i-1)"=w527:dbl[])  [unwired: 1 in, 1 out]
      n267 = Build Array(w527, w528) -> (w526:dbl[][])
      "elapsed time(s)" <- w526
      n268 = Index Array(array=w526, index (row)=0 ("指標 （行）")) -> (element=w524:dbl[])  [unwired: 1 in]
      n269 = Add Array Elements(numeric array=w524) -> (sum=→"Sumtime(s)":dbl)
    }
  }
